vi "parseForceAndStatusResponse.vi"(8 "error in (no error)":errorcluster, 10 "DynamicFrameParser":refnum<class "DynamicFrameParser.lvclass">, 11 "SAAILC in":refnum<class "SAAILC.lvclass">) -> (0 "error out":errorcluster, 3 "SAAILC out":refnum<class "SAAILC.lvclass">)   [LabVIEW 2016, in "RTFAILC.lvlib" / "SAAILC.lvclass"]
uses:
  SAAILC.lvclass
  D:/Code/Common_RT_FAILC/FAILC/FAILC.lvclass
  Common_RT_Modbus/DynamicFrameParser/DynamicFrameParser.lvclass
  Common_RT_Modbus/DataTypes/ExceptionCodes.ctl
  FAILC/FAILC.lvclass/FAILC.ctl
  FAILC/FAILC.lvclass
  Common_RT_Modbus/RTModbus.lvlib
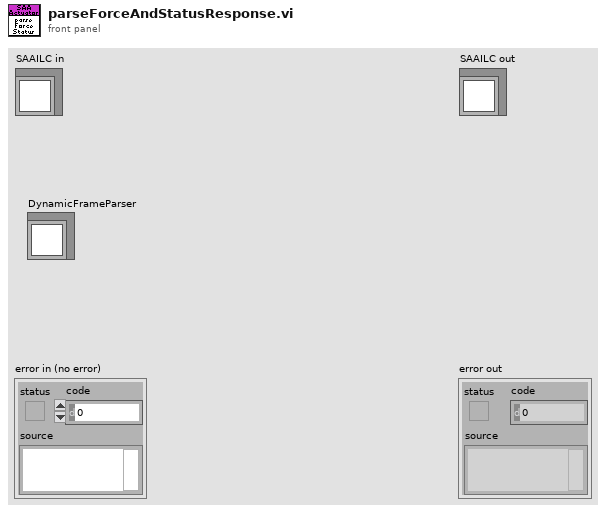
[diagram p1: front panel]
types:
  T1 = typedef "RTModbus.lvlib/ExceptionCodes.ctl" = u16
  T2 = typedef "RTFAILC.lvlib/FAData.ctl" = cluster{"Constants":T3, "Command":T4, "Telemetry":T6, "Responses":T7, "Timings":T8}
  T3 = typedef "RTFAILC.lvlib/FAConstants.ctl" = cluster{"ID":i16}
  T4 = typedef "RTFAILC.lvlib/FACommand.ctl" = cluster{"AxialSetPoint":i32, "LateralSetPoint":i32, "PressureServoValveSettings":T5, "BoosterValveSettings":T5}
  T5 = typedef "RTFAILC.lvlib/FAPID.ctl" = cluster{"Kp":sgl, "Ki":sgl, "Kd":sgl, "Kf":sgl}
  T6 = typedef "RTFAILC.lvlib/FATelemetry.ctl" = cluster{"ILCFault":bool, "BroadcastCounter":u8, "AxialLoadCellForce":sgl, "LateralLoadCellForce":sgl, "AxialPressure":T5, "AxialTurbo":T5, "LateralPressure":T5, "LateralTurbo":T5}
  T7 = typedef "RTFAILC.lvlib/FAResponses.ctl" = cluster{"PIDParameters":T1, "ReadPIDParameters":T1, "SetForce":T1, "ForceAndStatus":T1}
  T8 = typedef "RTFAILC.lvlib/FATimings.ctl" = cluster{"BroadcastSetForce":u32, "PIDParameters":u32, "FreezeSensorValues":u32, "ForceAndStatus":u32, "ReadPIDParameters":u32, "SetForce":u32}
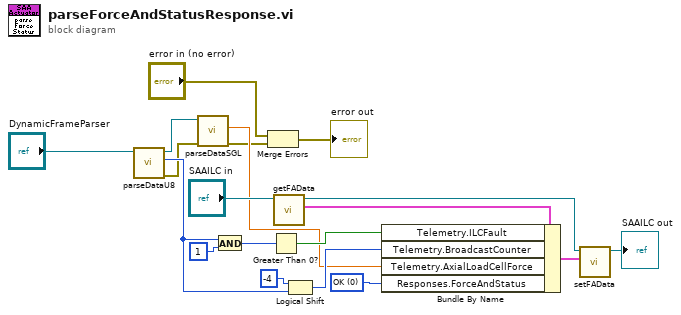
[diagram p0: block diagram]
diagram:
  w1 = T1 0 items=["OK", "IllegalFunction", "IllegalDataAddress", "IllegalDataValue", "SlaveDeviceFailure", "Acknowledge", "SlaveDeviceBusy", "NegativeAcknowledge", "MemoryParityError", "GatewayPathUnavailable", "GatewayTargetDeviceFailedToRespond"] ("FAResponses.ForceAndStatus")
  n1 = call "parseDataU8.vi"("FrameParser in"="DynamicFrameParser") -> ("error out"=w6:errorcluster, "Data"=w12:u8, "FrameParser out"=w8:refnum<class "DynamicFrameParser.lvclass">)  [unwired: 8 in]
  n2 = call "parseDataSGL.vi"("error in (no error)"=w6, "FrameParser in"=w8) -> ("error out"=w5:errorcluster, "Data"=w9:sgl)  [unwired: 7 in, 1 out]
  n3 = And(x=w12, y=u8 1) -> (x .and. y?=w14:u8)
  n4 = Merge Errors("error in (no error)", w5) -> (→"error out":errorcluster)
  n5 = Greater Than 0?(x=w14) -> (x > 0?=w13:bool)
  n6 = call "getFAData.vi"("FAILC in"="SAAILC in") -> ("FAData"=w18:T2, "FAILC out"=w16:refnum<class "SAAILC.lvclass">)  [unwired: 9 in]
  n7 = Logical Shift(y=i16 -4, x=w12) -> (x << y=w10:u8)
  n8 = Bundle By Name(cluster=w18, "Telemetry.ILCFault"=w13, "Telemetry.BroadcastCounter"=w10, "Telemetry.AxialLoadCellForce"=w9, "Responses.ForceAndStatus"=w1) -> (w17:T2)
  n9 = call "setFAData.vi"("FAData"=w17, "FAILC in"=w16) -> ("FAILC out"=→"SAAILC out":refnum<class "SAAILC.lvclass">)  [unwired: 9 in]
